vi "BuildTestFromLibrary.vi"(8 "error in (no error)":errorcluster, 10 "Library Refnum":refnum<vi>, 11 "LVUnitTestBuilder in":refnum<class "LVUnitTestBuilder.lvclass">) -> (0 "error out":errorcluster, 2 "Test":refnum<class "Test.lvclass">, 3 "LVUnitTestBuilder out":refnum<class "LVUnitTestBuilder.lvclass">)   [LabVIEW 2019, in "LVUnitTestBuilder.lvclass"]
uses:
  LVUnitTestBuilder.lvclass
  Test/Test.lvclass
  TestSuite/TestSuite.lvclass
  C:/Users/de200256/Code/neuperger/lvunit/Test/Test.lvclass
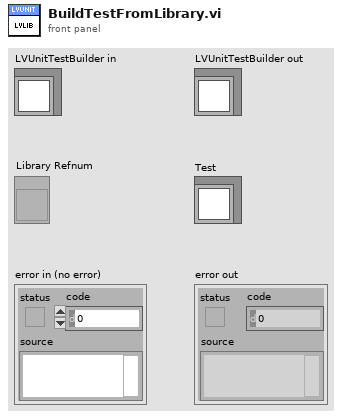
[diagram p1: front panel]
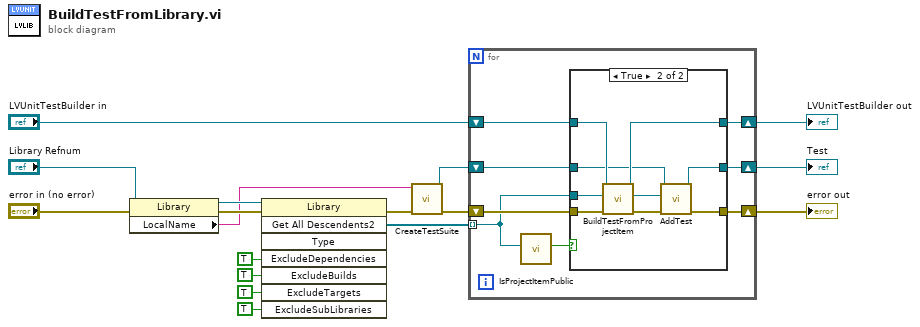
[diagram p0: block diagram]
diagram:
  n1 = property class="Library"(reference="Library Refnum", error in="error in (no error)") -> (reference out=w4:refnum<vi>, error out=w6:errorcluster, "LocalName"=w2:string)
  n2 = invoke class="Library" method="Get All Descendents2"(reference=w4, error in=w6, "ExcludeDependencies"=TRUE, "ExcludeBuilds"=TRUE, "ExcludeTargets"=TRUE, "ExcludeSubLibraries"=TRUE) -> (error out=w10:errorcluster, "Get All Descendents2"=w12:refnum<vi>[])  [unwired: 2 in, 6 out]
  n3 = call "CreateTestSuite.vi"("error in (no error)"=w10, "Name"=w2) -> ("error out"=w3:errorcluster, "TestSuite"=w1:refnum<class "TestSuite.lvclass">)  [unwired: 8 in]
  n4 = for {
    tunnel: w12 -> [w19] mode=indexing
    shift-right: [w22] -> w11
    shift-left: w3 -> [w25]
    shift-right: [w23] -> w8
    shift-left: "LVUnitTestBuilder in" -> [w24]
    shift-right: [w21] -> w7
    shift-left: w1 -> [w20]
    n5 = call "IsProjectItemPublic.vi"("ProjectItem Refnum"=w19) -> ("Is Public"=w18:bool)  [unwired: 10 in]
    n6 = case shown="True" w18 {
      tunnel: w25 -> [w28 w37]
      tunnel: w24 -> [w26 w35]
      tunnel: [w26 w34] -> w23
      tunnel: [w28 w33] -> w22
      tunnel: [w27 w31] -> w21
      tunnel: w20 -> [w27 w30]
      tunnel: w19 -> [_ w29]
      frame False {
        # "Skip non-public members"
      }
      frame True {
        n7 = call-dynamic "BuildTestFromProjectItem.vi"("error in (no error)"=w37, "ProjectItem Refnum"=w29, "LVUnitTestBuilder in"=w35) -> ("error out"=w36:errorcluster, "Test"=w32:refnum<class "Test.lvclass">, "LVUnitTestBuilder out"=w34:refnum<class "LVUnitTestBuilder.lvclass">)  [unwired: 6 in]
        n8 = call-dynamic "AddTest.vi"("error in (no error)"=w36, "Test"=w32, "TestSuite in"=w30) -> ("error out"=w33:errorcluster, "TestSuite out"=w31:refnum<class "TestSuite.lvclass">)  [unwired: 7 in]
      }
    }
  }
  "error out" <- w11
  "LVUnitTestBuilder out" <- w8
  "Test" <- w7
